vi "initialize_lib_tsmaster.vi"(8 "error in (no error)":errorcluster caption="Incorrect input (no errors)", 10 "AppName":string="LABFD", 11 "Path input":path) -> (0 "error output":errorcluster, 3 "Path output":path)   [LabVIEW 2014]
doc: "Call location:\nBefore using TsMasterApi, the module initialization function must be executed to initialize the internal parameters\nNumber, prepare the environment for driving operation.\ninput parameter : \nAAppName: Application name, cannot be empty. Hardware channel parameters are all bound to this name.\nUsers can input the set string, such as \"TestDemo\", or directly obtain it through the following statement\nTake the name of the current application,\nAnd pass it as a parameter to initialize this API module:\nSystem.IO.Path.GetFileNameWithoutExtension(System. Windows.Forms.Appl ication.ExecutablePath)"
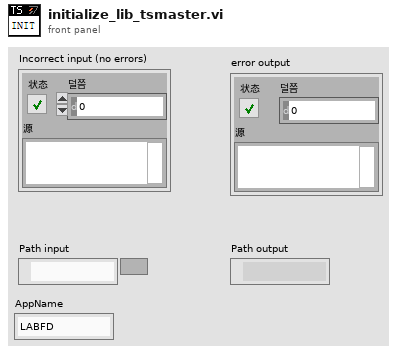
[diagram p1: front panel]
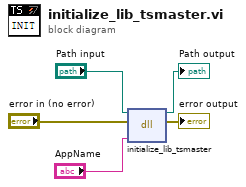
[diagram p0: block diagram]
diagram:
  n1 = dll-call lib="PTH2Habs CUsers\nAdministratorDesktopTS_Can通讯PathTSMaster.dll" fn="initialize_lib_tsmaster"(path in="Path input", error in="error in (no error)", "AppName"="AppName") -> (path out=→"Path output":path, error out=→"error output":errorcluster)  [unwired: 3 in]
